vi "channel settings to type and function support.vi"(8 "error in":errorcluster, 11 "FixedChannelTBModuleDecideFeatures in":refnum<class "FixedChannelTBModuleDecideFeatures.lvclass">) -> (0 "error out":errorcluster, 3 "FixedChannelTBModuleDecideFeatures out":refnum<class "FixedChannelTBModuleDecideFeatures.lvclass">)   [LabVIEW 2013, in "FixedChannelTBModuleDecideFeatures.lvclass"]
uses:
  FixedChannelTBModuleDecideFeatures.lvclass
  <vilib>/NI/Tag Bus/tag/Data Type.ctl
  FixedChannelTBModuleDecideFeatures.lvclass/FixedChannelTBModuleDecideFeatures.ctl
  <vilib>/NI/Tag Bus Module Framework/channel/channel classification.ctl
  <vilib>/NI/Tag Bus/tag/tag descriptor.lvclass
  <vilib>/NI/Tag Bus Module Framework/channel/TBM channel.lvclass
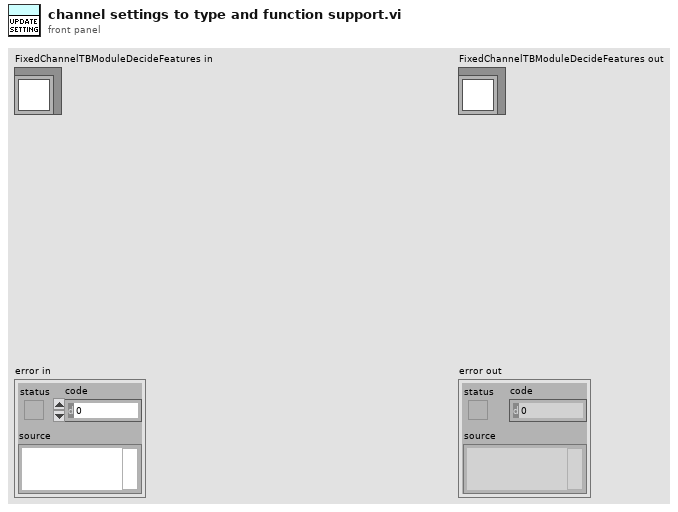
[diagram p1: front panel]
types:
  T1 = typedef "tag bus.lvlib/tag descriptor.lvclass/Data Type.ctl" = enum16{"Double", "Single", "I64", "I32", "I16", "I8", "U64", "U32", "U16", "U8", "Boolean", "String", "Array of Double", "Array of Single", "Array of I64", "Array of I32", "Array of I16", "Array of I8", "Array of U64", "Array of U32", "Array of U16", "Array of U8", "Array of Boolean", "Array of String"}
  T2 = typedef "FixedChannelTBModuleDecideFeatures.lvclass/channel configuration.ctl" = cluster{"Name":string, "channel classification":T3, "data type":T1}
  T3 = typedef "TBM channel.lvclass/channel classification.ctl" = enum16{"input data", "output data", "processing parameter", "processing result"}
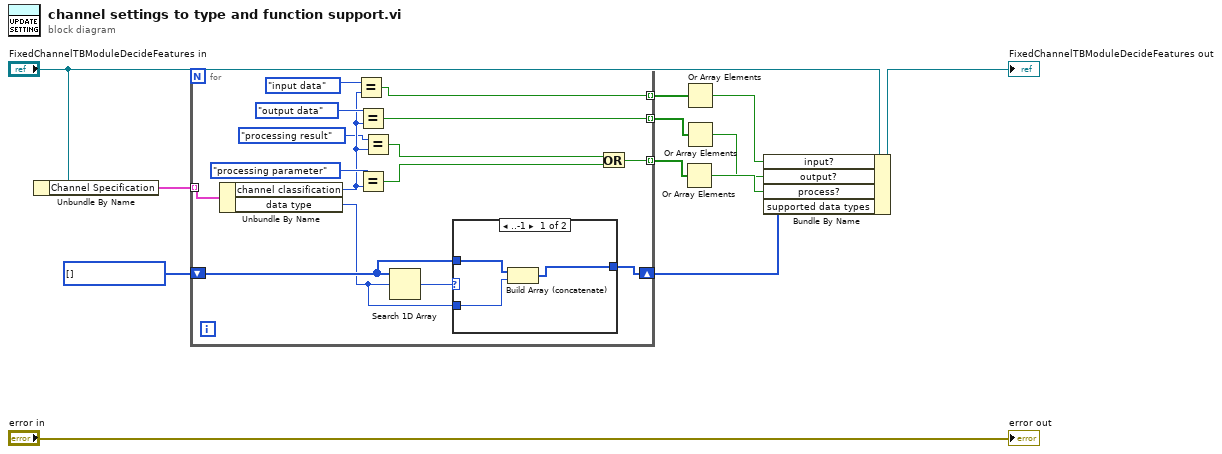
[diagram p0: block diagram]
diagram:
  w8 = T1[] [] items=["Double", "Single", "I64", "I32", "I16", "I8", "U64", "U32", "U16", "U8", "Boolean", "String", "Array of Double", "Array of Single", "Array of I64", "Array of I32", "Array of I16", "Array of I8", "Array of U64", "Array of U32", "Array of U16", "Array of U8", "Array of Boolean", "Array of String"] ("supported data types")
  n1 = Unbundle By Name("FixedChannelTBModuleDecideFeatures in") -> ("Channel Specification"=w9:T2[])
  n2 = for {
    tunnel: w9 -> [w27] mode=indexing
    shift-right: [w15] -> w7
    shift-left: w8 -> [w14]
    tunnel: [w19] -> w6 mode=indexing
    tunnel: [w18] -> w5 mode=indexing
    tunnel: [w17] -> w4 mode=indexing
    n3 = Unbundle By Name(w27) -> ("channel classification"=w23:T3, "data type"=w13:T1)
    n4 = Equal?(x=channel_classification."input data", y=w23) -> (x = y?=w19:bool)
    n5 = Equal?(x=channel_classification."output data", y=w23) -> (x = y?=w18:bool)
    n6 = Equal?(x=channel_classification."processing parameter", y=w23) -> (x = y?=w21:bool)
    n7 = Equal?(x=channel_classification."processing result", y=w23) -> (x = y?=w20:bool)
    n8 = Search 1D Array(1D array=w14, element=w13) -> (index of element=w16:i32)  [unwired: 1 in]
    n9 = case shown="..-1" w16 {
      tunnel: [w28 w31] -> w15
      tunnel: w14 -> [w30 w31]
      tunnel: w13 -> [w29 _]
      frame ..-1 {
        n10 = Build Array (concatenate)(w30, w29) -> (w28:T1[])
      }
      frame 0.. {
      }
    }
    n11 = Or(x=w20, y=w21) -> (x .or. y?=w17:bool)
  }
  n12 = Or Array Elements(Boolean array=w4) -> (logical OR=w3:bool)
  n13 = Or Array Elements(Boolean array=w6) -> (logical OR=w1:bool)
  n14 = Or Array Elements(Boolean array=w5) -> (logical OR=w2:bool)
  n15 = Bundle By Name(cluster="FixedChannelTBModuleDecideFeatures in", "input?"=w1, "output?"=w2, "process?"=w3, "supported data types"=w7) -> (→"FixedChannelTBModuleDecideFeatures out":refnum<class "FixedChannelTBModuleDecideFeatures.lvclass">)
  "error out" <- "error in"
